vi "About_equal.vi"(10 "B":dbl, 11 "A":dbl) -> (3 "About equal":bool)   [LabVIEW 2017]
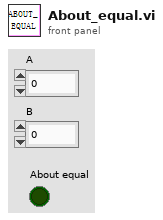
[diagram p1: front panel]
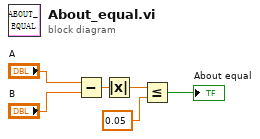
[diagram p0: block diagram]
diagram:
  n1 = Subtract(x="A", y="B") -> (x-y=w4:dbl)
  n2 = Absolute Value(x=w4) -> (abs(x)=w3:dbl)
  n3 = Less Or Equal?(x=w3, y=0.05) -> (x <= y?=→"About equal":bool)
